vi "Open KH7008.vi"(8 "error in (no error)":errorcluster) -> (0 "error out":errorcluster)   [LabVIEW 2019, in "Control Experiment.lvclass"]
uses:
  Control Experiment.lvclass
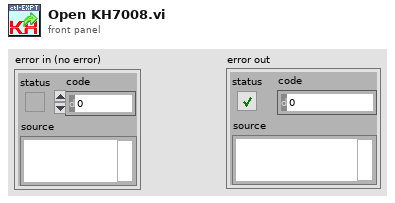
[diagram p1: front panel]
types:
  T1 = enum32{"Invalid", "Standard", "Closed", "Hidden", "Minimized", "Maximized"}
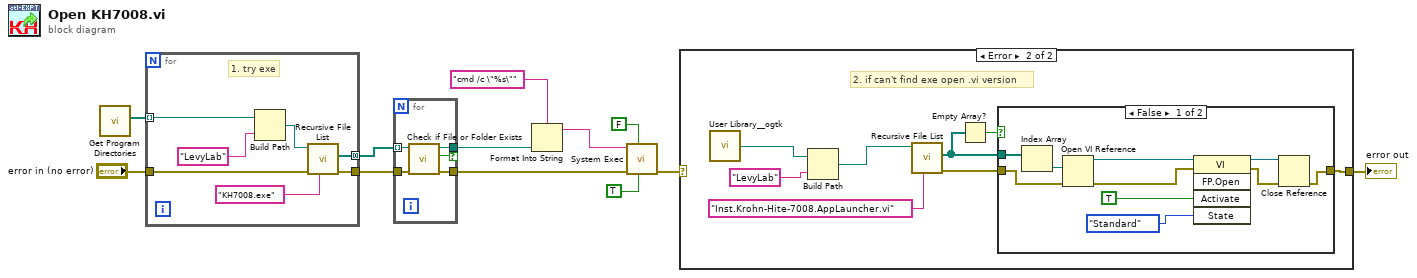
[diagram p0: block diagram]
diagram:
  n1 = call "Get Program Directories.vi"() -> ("Program Directories"=w8:path[])  [unwired: 11 in]
  n2 = for {
    tunnel: w8 -> [w15] mode=indexing
    tunnel: "error in (no error)" -> [w17]
    tunnel: [w14] -> w7
    tunnel: [w13] -> w6 mode=concatenating
    # "1. try exe"
    n3 = Build Path(base path=w15, name or relative path="LevyLab") -> (appended path=w19:path)
    n4 = call <vilib>:"Recursive File List.vi"("pattern"="KH7008.exe", "error in (no error)"=w17, "Folder Path"=w19) -> ("error out"=w14:errorcluster, "All Files in Dir"=w13:path[])  [unwired: 4 in, 3 out]
  }
  n5 = for {
    tunnel: w7 -> [w24]
    tunnel: w6 -> [w23] mode=indexing
    tunnel: [w22] -> w3 if=w21
    tunnel: [w20] -> w5
    n6 = call <vilib>:"Check if File or Folder Exists.vi"("error in (no error)"=w24, "path"=w23) -> ("error out"=w20:errorcluster, "file or folder exists?"=w21:bool, "dup path"=w22:path)  [unwired: 7 in]
  }
  n7 = Format Into String(format string="cmd /c \"%s\"", w3) -> (resulting string=w2:string)  [unwired: 2 in, 1 out]
  n8 = call <vilib>:"System Exec.vi"("run minimized? (F)"=TRUE, "wait until completion? (T)"=FALSE, "error in (no error)"=w5, "command line"=w2) -> ("error out"=w11:errorcluster)  [unwired: 4 in, 3 out]
  n9 = case shown="Error" w11 {
    selector: w11 -> [w25 _]
    tunnel: [w25 w29] -> w10
    frame No Error {
    }
    frame Error {
      # "2. if can't find exe open .vi version"
      n10 = call <userlib>:"User Library__ogtk.vi"() -> ("User Library (+ Relative)"=w27:path)  [unwired: 1 in]
      n11 = Build Path(base path=w27, name or relative path="LevyLab") -> (appended path=w26:path)
      n12 = call <vilib>:"Recursive File List.vi"("pattern"="Inst.Krohn-Hite-7008.AppLauncher.vi", "Folder Path"=w26) -> ("error out"=w30:errorcluster, "All Files in Dir"=w31:path[])  [unwired: 5 in, 3 out]
      n13 = Empty Array?(array=w31) -> (empty?=w32:bool)
      n14 = case shown="False" w32 {
        tunnel: w31 -> [w36 _]
        tunnel: w30 -> [w35 w44]
        tunnel: [w34 w44] -> w29
        frame False {
          n15 = Index Array(array=w36) -> (element=w37:path)  [unwired: 1 in]
          n16 = Open VI Reference(vi path=w37, error in (no error)=w35) -> (vi reference=w38:refnum<vi>, error out=w43:errorcluster)  [unwired: 4 in]
          n17 = invoke class="VI" method="FP.Open"(reference=w38, error in=w43, "Activate"=TRUE ("Activate?"), "State"=T1."Standard") -> (reference out=w39:refnum<vi>, error out=w40:errorcluster)  [unwired: 1 in, 3 out]
          n18 = Close Reference(reference=w39, error in (no error)=w40) -> (error out=w34:errorcluster)
        }
        frame True {
        }
      }
    }
  }
  "error out" <- w10
